vi "Add to Cache.vi"(8 "error in (no error)":errorcluster, 10 "Topic":string, 11 "TopicFilter in":refnum<class "_TopicFilter.lvclass">) -> (0 "error out":errorcluster, 1 "added to cache":bool, 3 "TopicFilter out":refnum<class "_TopicFilter.lvclass">)   [LabVIEW 2013, in "MQTT Server.lvlib" / "_TopicFilter.lvclass"]
uses:
  _TopicFilter.lvclass
  _TopicFilter.lvclass/_TopicFilter.ctl
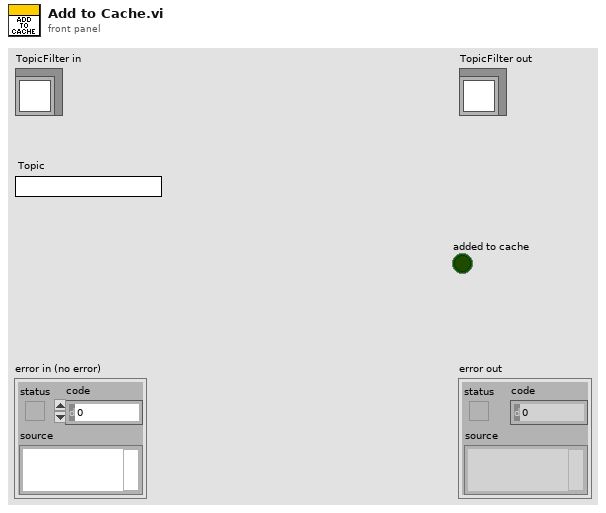
[diagram p1: front panel]
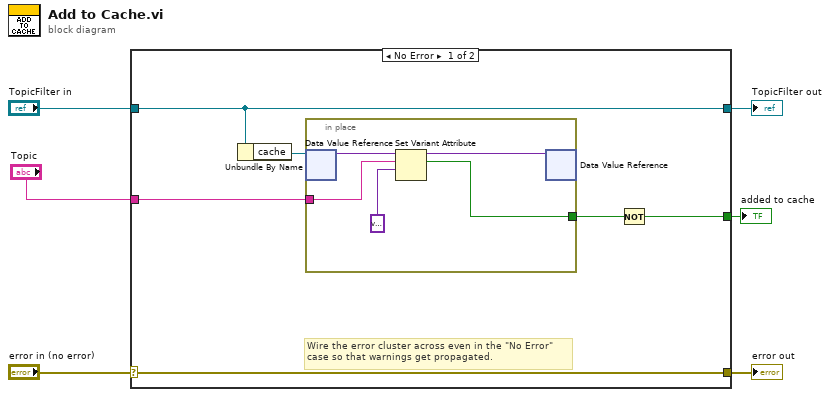
[diagram p0: block diagram]
diagram:
  n1 = case shown="No Error" "error in (no error)" {
    selector: "error in (no error)" -> [w12 w19]
    tunnel: [w12 w19] -> w5
    tunnel: [w11 w18] -> w3
    tunnel: "TopicFilter in" -> [w11 w18]
    tunnel: "Topic" -> [w9 _]
    tunnel: [w7 _] -> w1
    frame No Error {
      # "Wire the error cluster across even in the \"No Error\"\ncase so that warnings get propagated."
      n2 = Unbundle By Name(w11) -> ("cache"=w10:refnum<data-value>)
      n3 = in-place {
        in-place-border: w9 -> [w15]
        in-place-border: [w13] -> w8
        n4 = in-place-dvr #1(w10) -> (w17:variant)  [unwired: 1 out]
        n5 = Set Variant Attribute(Variant=w17, name=w15, value=variant ("variant")) -> (Variant out=w16:variant, replaced=w13:bool)  [unwired: 1 in, 1 out]
        n6 = in-place-dvr #1(w16) -> ()  [unwired: 2 out]
      }
      n7 = Not(x=w8) -> (.not. x?=w7:bool)
    }
    frame Error {
    }
  }
  "error out" <- w5
  "TopicFilter out" <- w3
  "added to cache" <- w1
